vi "View.vi"(8 "error in (no error)":errorcluster, 11 "View In":refnum<class "View.lvclass">) -> (0 "error out":errorcluster)   [LabVIEW 2020, in "View.lvclass"]
doc: "This VI implements the main UI of the process. A reference to this VI should be set using the Set View VI Reference.vi method when the VI is started."
uses:
  View.lvclass
  C:/git/astemes-triarc-framework/source/Framework/Process/Process.lvclass
  View.lvclass/View.ctl
  Process/Process.lvclass
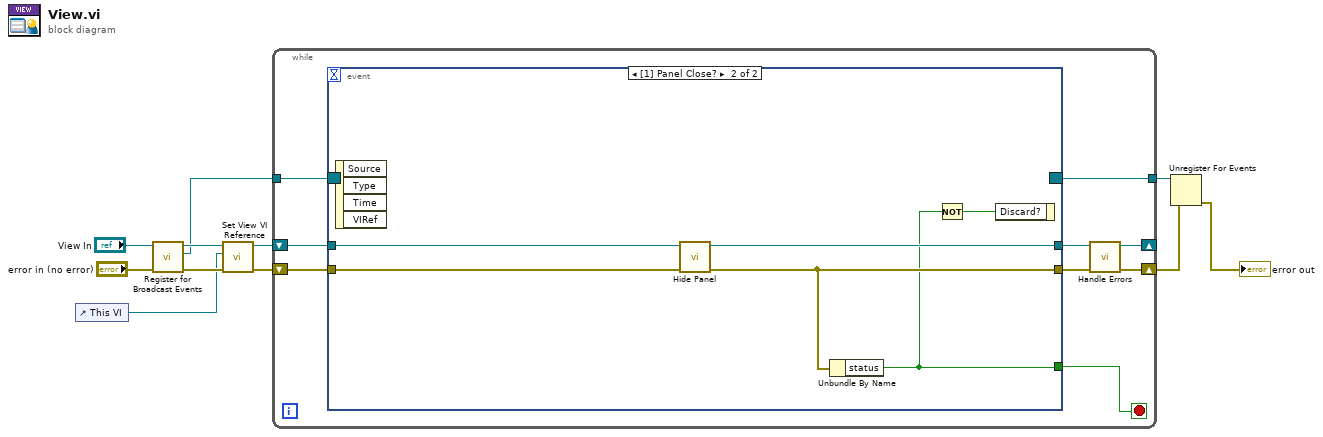
[diagram p0: block diagram]
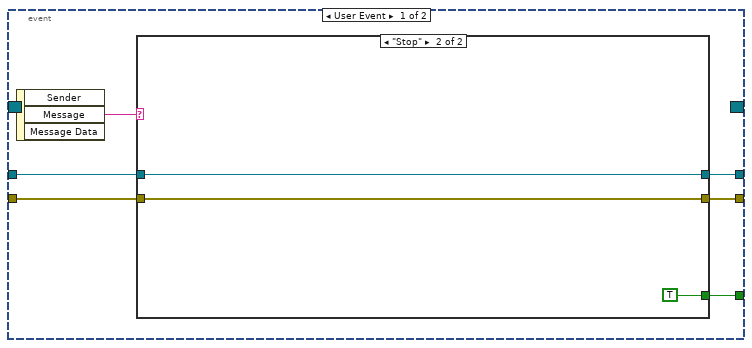
[diagram p2: hidden frame]
diagram:
  n1 = control-ref of="This VI"() -> (w1:refnum<vi>)
  n2 = call "Register for Broadcast Events.vi"("error in (no error)"="error in (no error)", "Process In"="View In") -> ("error out"=w3:errorcluster, "Event Registration Refnum Out"=w2:refnum<event-registration>, "Process Out"=w5:refnum<class "View.lvclass">)  [unwired: 7 in]
  n3 = call "Set View VI Reference.vi"("error in (no error)"=w3, "View VI Reference"=w1, "View In"=w5) -> ("error out"=w8:errorcluster, "View Out"=w9:refnum<class "View.lvclass">)  [unwired: 7 in]
  n4 = while {
    shift-right: [w14] -> _
    shift-left: w9 -> [w20]
    shift-right: [w12] -> w10
    shift-left: w8 -> [w18]
    tunnel: w2 -> [w17]
    tunnel: [w16] -> w11
    stop <- w15 stop-if-true
    n5 = event shown="[1] Panel Close?" {
      selector: w17 -> [_ _]
      dyn-events: [_ _] -> w16
      timeout: _ -> [_ _]
      tunnel: w20 -> [w26 w36]
      tunnel: [w25 w35] -> w19
      tunnel: w18 -> [w23 w37]
      tunnel: [w24 w34] -> w13
      tunnel: [w21 w32] -> w15
      event User Event {
        n6 = event-data() -> ("Message"=w22:string)  [unwired: 1 in, 2 out]
        n7 = case shown="\"Stop\"" w22 {
          tunnel: w26 -> [w28 w31]
          tunnel: [w28 w31] -> w25
          tunnel: [w27 w30] -> w24
          tunnel: w23 -> [w27 w30]
          tunnel: [_ TRUE] -> w21
          frame Default {
          }
          frame "Stop" {
          }
        }
      }
      event Panel Close? {
        n8 = event-data() -> ()  [unwired: 1 in, 4 out]
        n9 = call "Hide Panel.vi"("error in (no error)"=w37, "View In"=w36) -> ("error out"=w34:errorcluster, "View Out"=w35:refnum<class "View.lvclass">)  [unwired: 8 in]
        n10 = Unbundle By Name(w34) -> ("status"=w32:bool)
        n11 = Not(x=w32) -> (.not. x?=w33:bool)
        n12 = event-data("Discard?"=w33) -> ()  [unwired: 1 in, 1 out]
      }
    }
    n13 = call-dynamic "Handle Errors.vi"("error in (no error)"=w13, "Process In"=w19) -> ("error out"=w12:errorcluster, "Process Out"=w14:refnum<class "View.lvclass">)  [unwired: 8 in]
  }
  n14 = Unregister For Events(event registration refnum=w11, error in=w10) -> (error out=→"error out":errorcluster)
